vi "LAB1_ex4.vi"() -> ()   [LabVIEW 2015]
doc: "This example demonstrates how to read N channels of analog input from a LINX device."
uses:
  <vilib>/MakerHub/LINX/Public/Peripherals/PWM/PWM Set Duty Cycle 1 Chan.vi
  <vilib>/MakerHub/LINX/Public/Utilities/Open Serial.vi
  <vilib>/MakerHub/LINX/Public/Peripherals/PWM/PWM Set Duty Cycle N Chans.vi
  <vilib>/MakerHub/LINX/LMH-LINX.lvlib
panel:
  out "Duty Cycle":dbl(graph)
  out "Vout":dbl(graph)
  in  "Temperature":dbl
  in  "Humidity":dbl
  in  "Stop Button":bool
  in  "Serial Port":refnum<visa-resource-name>
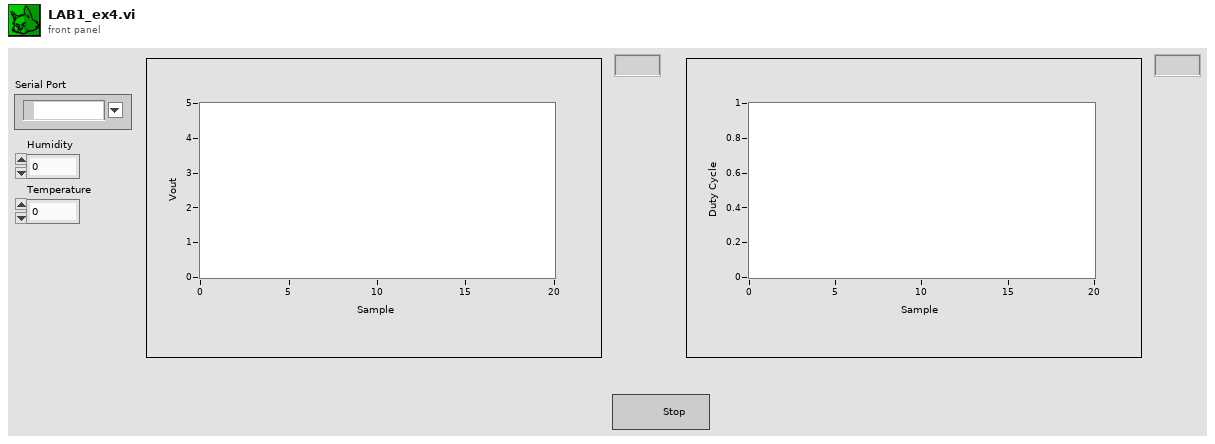
[diagram p1: front panel]
types:
  T1 = typedef "LMH-LINX.lvlib/LINX Ref.ctl" = cluster{"IO":T2, "Interface":T3, "LINX Device Config":T4}
  T2 = typedef "LMH-LINX.lvlib/Platform.ctl" = enum16{"Remote", "Local"}
  T3 = typedef "LMH-LINX.lvlib/Interface.ctl" = enum16{"Serial", "TCP"}
  T4 = typedef "LMH-LINX.lvlib/Device.lvlib/LINX Device Config.ctl" = cluster{"Interface":T3, "COM Port":refnum<visa-resource-name>, "TCP Configuration":T5, "Device Family":u8, "Device ID":u8, "Device Name":string, "TCP Ref":refnum<k5>, "Channels":T6}
  T5 = typedef "LMH-LINX.lvlib/Device.lvlib/TCP Config.ctl" = cluster{"IP Address":string, "Port":u16}
  T6 = typedef "LMH-LINX.lvlib/Channels.ctl" = cluster{"DI":u8[], "DO":u8[], "AI":u8[], "AO":u8[], "PWM":u8[], "QE":u8[], "UART":u8[], "I2C 2":u8[], "SPI":u8[], "CAN":u8[], "Servo":u8[], "AI Ref (V)":dbl, "AI Resolution (Bits)":u8, "AO Ref (V)":dbl, "AO Resolution (Bits)":u8}
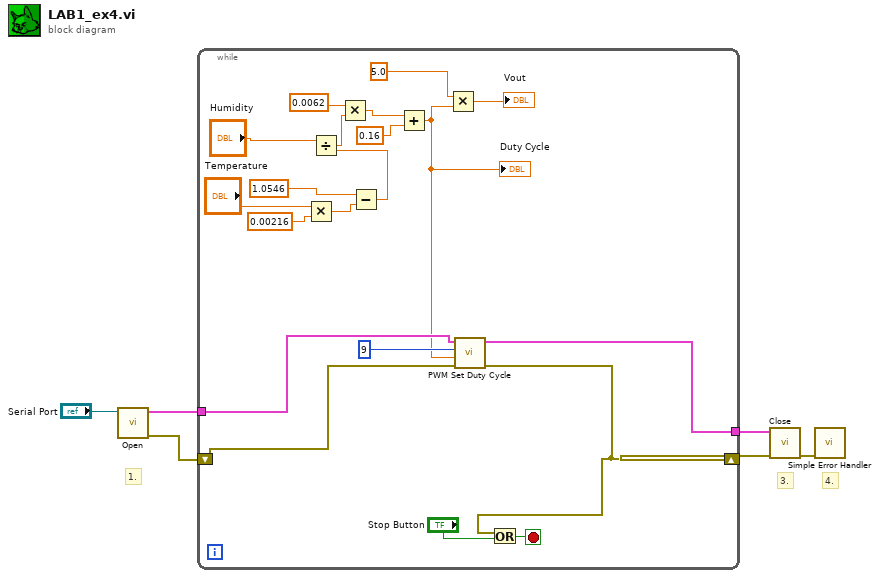
[diagram p0: block diagram]
diagram:
  # "4."
  # "3."
  # "1."
  n1 = call-poly <vilib>:"Open.vi"("Serial Port"="Serial Port") -> ("Error Out"=w5:errorcluster, "LINX Resource"=w6:T1)  [unwired: 8 in, 1 out]
  n2 = while {
    tunnel: w6 -> [w9]
    shift-right: [w10] -> w4
    shift-left: w5 -> [w11]
    tunnel: [w8] -> w1
    stop <- w26 stop-if-true
    n3 = Multiply(x="Temperature", y=0.00216) -> (x*y=w22:dbl)
    n4 = Subtract(x=1.0546, y=w22) -> (x-y=w20:dbl)
    n5 = Divide(x="Humidity", y=w20) -> (x/y=w18:dbl)
    n6 = Multiply(x=0.0062, y=w18) -> (x*y=w16:dbl)
    n7 = Add(x=w16, y=0.16) -> (x+y=w7:dbl)
    "Duty Cycle" <- w7
    n8 = Multiply(x=5.0, y=w7) -> (x*y=→"Vout":dbl)
    n9 = call-poly <vilib>:"PWM Set Duty Cycle.vi"("Error In"=w11, "Duty Cycle (0-1)"=w7, "PWM Channel"=9, "LINX Resource"=w9) -> ("Error Out"=w10:errorcluster, "LINX Resource"=w8:T1)  [unwired: 6 in]
    n10 = Or(x=w10, y="Stop Button") -> (x .or. y?=w26:bool)
  }
  n11 = call <vilib>:"Close.vi"("Error In"=w4, "LINX Resource"=w1) -> ("Error Out"=w2:errorcluster)  [unwired: 9 in]
  n12 = call <vilib>:"Simple Error Handler.vi"("error in (no error)"=w2) -> ()  [unwired: 4 in, 5 out]
